vi "sub_USRP_init_Tx.vi"(10 "Tx Parameters":T1={"IQ rate (Hz)"=200000.0, "Carrier frequency [Hz]"=1187500000.0, "Gain [dB]"=16.0, "Tx device name"="192.168.10.2; 192.168.10.3;"} {"Gain [dB]" format="%#_6f"; "Carrier frequency [Hz]" format="%#_6p"; "IQ rate (Hz)" format="%#_6p"}) -> (0 "Error out":errorcluster, 3 "Tx Session handle out":refnum<k15>="192.168.10.2 (5)")   [LabVIEW 2012]
uses:
  <instrlib>/niUSRP/niUSRP Timestamp.ctl
  <instrlib>/niUSRP/niUSRP Configure Time Start Trigger.vi
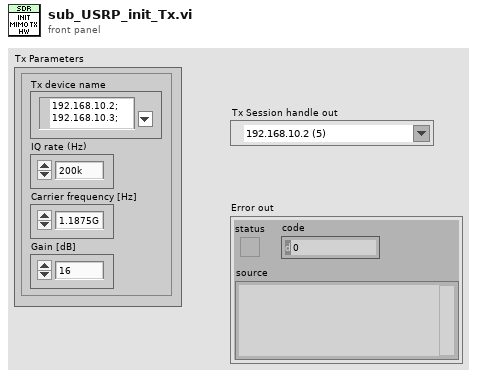
[diagram p1: front panel]
types:
  T1 = cluster{"IQ rate (Hz)":dbl, "Carrier frequency [Hz]":dbl, "Gain [dB]":dbl, "Tx device name":refnum<k15>}
  T2 = typedef "niUSRP Timestamp.ctl" = cluster{"whole seconds":u64, "fractional seconds":dbl}
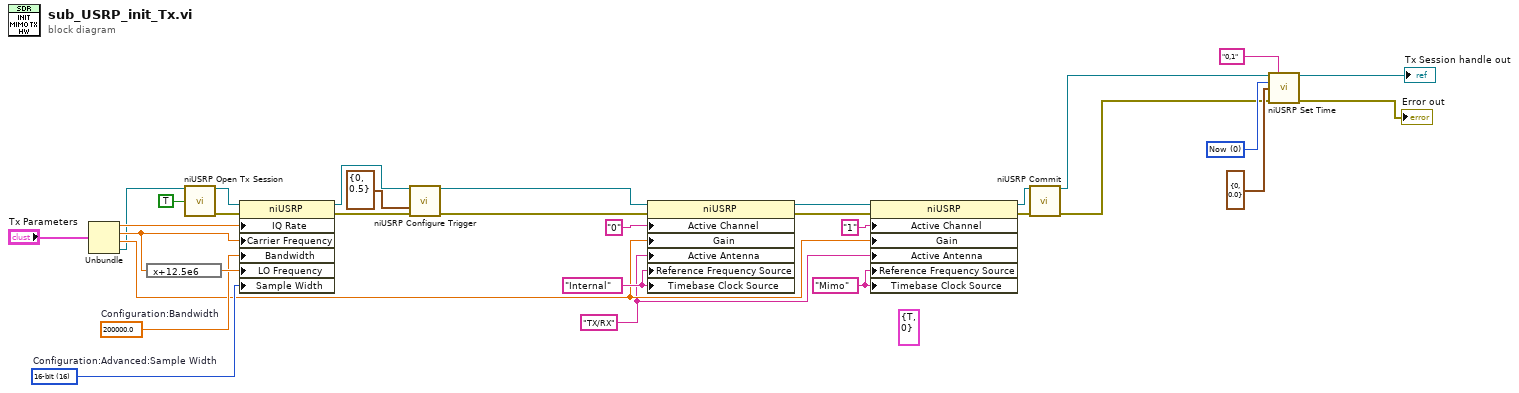
[diagram p0: block diagram]
diagram:
  w1 = "TX/RX" ("Configuration:Active Antenna")
  w9 = 0 items=["Now", "Next Timebase Edge"] ("apply timestamp")
  w19 = "Mimo" ("Clocking and Synchronization:Reference Frequency Source")
  (unwired) cluster{"status":bool, "code":i32} {"status"=TRUE, "code"=0} ("error in")
  w27 = 200000.0  # Configuration:Bandwidth
  w26 = 16 items=["16-bit"=16, "8-bit"=8]  # Configuration:Advanced:Sample Width
  w24 = "Internal" ("Clocking and Synchronization:Reference Frequency Source")
  n1 = Unbundle("Tx Parameters") -> ("IQ rate (Hz)"=w30:dbl, "Carrier frequency [Hz]"=w29:dbl, "Gain [dB]"=w20:dbl, "Tx device name"=w2:refnum<k15>)
  n2 = expression code="x+12.5e6"(w29) -> (w28:dbl)
  n3 = call <instrlib>:"niUSRP Open Tx Session.vi"("device names"=w2, "reset"=TRUE) -> ("session handle out"=w18:refnum<k15>, "error out"=w17:errorcluster)  [unwired: 12 in]
  n4 = property class="niUSRP"(reference=w18, error in=w17, "IQ Rate"=w30, "Carrier Frequency"=w29, "Bandwidth"=w27, "LO Frequency"=w28, "Sample Width"=w26) -> (reference out=w16:refnum<k15>, error out=w15:errorcluster)
  n5 = call-poly <instrlib>:"niUSRP Configure Trigger.vi"("session handle"=w16, "start trigger time"=T2 {"whole seconds"=0, "fractional seconds"=0.5}, "error in (no error)"=w15) -> ("session handle out"=w14:refnum<k15>, "error out"=w13:errorcluster)  [unwired: 11 in]
  n6 = property class="niUSRP"(reference=w14, error in=w13, "Active Channel"="0", "Gain"=w20, "Active Antenna"=w1, "Reference Frequency Source"=w24, "Timebase Clock Source"=w24) -> (reference out=w22:refnum<k15>, error out=w21:errorcluster)
  n7 = property class="niUSRP"(reference=w22, error in=w21, "Active Channel"="1", "Gain"=w20, "Active Antenna"=w1, "Reference Frequency Source"=w19, "Timebase Clock Source"=w19) -> (reference out=w11:refnum<k15>, error out=w12:errorcluster)
  n8 = call <instrlib>:"niUSRP Commit.vi"("session handle"=w11, "error in (no error)"=w12) -> ("session handle out"=w6:refnum<k15>, "error out"=w5:errorcluster)  [unwired: 12 in]
  n9 = call <instrlib>:"niUSRP Set Time.vi"("session handle"=w6, "channel list"="0,1", "apply timestamp"=w9, "timestamp"=T2 {"whole seconds"=0, "fractional seconds"=0.0}, "error in (no error)"=w5) -> ("session handle out"=→"Tx Session handle out":refnum<k15>, "error out"=→"Error out":errorcluster)  [unwired: 9 in]
